vi "NXT Camera Test8.vi"() -> ()   [LabVIEW 2016]
uses:
  <vilib>/NXT/Block Support/NXT_InputPort.ctl
  <vilib>/NXT/Block Support/NXT_OutputPort.ctl
  <vilib>/NXT/Dual Mode Library/Sensors/EV3_Ultrasonic_CM.vi
  <vilib>/NXT/NXTIO Xnodes/NXTIONodeSubVIs/NXTMoveMotors.vi
  <vilib>/NXT/NXTIO Xnodes/NXTIONodeSubVIs/NXTStopMotors.vi
  <vilib>/NXT/Subs/LVHSConnector.ctl
  <vilib>/NXT/NXTIO Xnodes/AddressXNode/NXTIOAddress.xnode
  <vilib>/NXT/NXTIO Xnodes/NXTIOXNode/NXTIO.xnode
  <vilib>/NXT/LegoClasses/BrickReference/BrickReference.lvclass
panel:
  out "Power":bool
  out "X Upper Left":u8
  out "X Lower Right":u8
  out "Y Lower Right":u8
  out "Y Upper Left":u8
  out "Count":u8
  out "Color":u8
  in  "Cluster":T1 {"Tracking Mode" items=["Disable Tracking", "Get First Object", "Get n th Object", "Enable Tracking", "Sort Objects  by size", "Sort Objects  by Colors", "Illumination on ", "Illumination Off", "Write Colormap", "Read Colormap", "Line tracking mode", "Object Tracking mode"]}
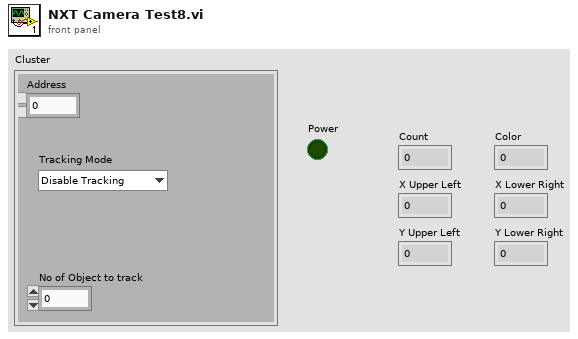
[diagram p1: front panel]
types:
  T1 = cluster{"Address":dbl, "No of Object to track":dbl, "Tracking Mode":u8}
  T2 = cluster{"Tracking Mode":u8, "Object Number to Track":u8, "Address":u8}
  T3 = typedef "NXT_InputPort.ctl" = u32
  T4 = typedef "LVHSConnector.ctl" = refnum<class "BrickReference.lvclass">
  T5 = typedef "NXT_OutputPort.ctl" = u8
  T6 = cluster{"Total Tracked Objects":u8, "Color":u8, "X Upper Left":u8, "Y Upper Left":u8, "X Lower Right":u8, "Y Lower Right":u8, "Status (boolean)":bool}
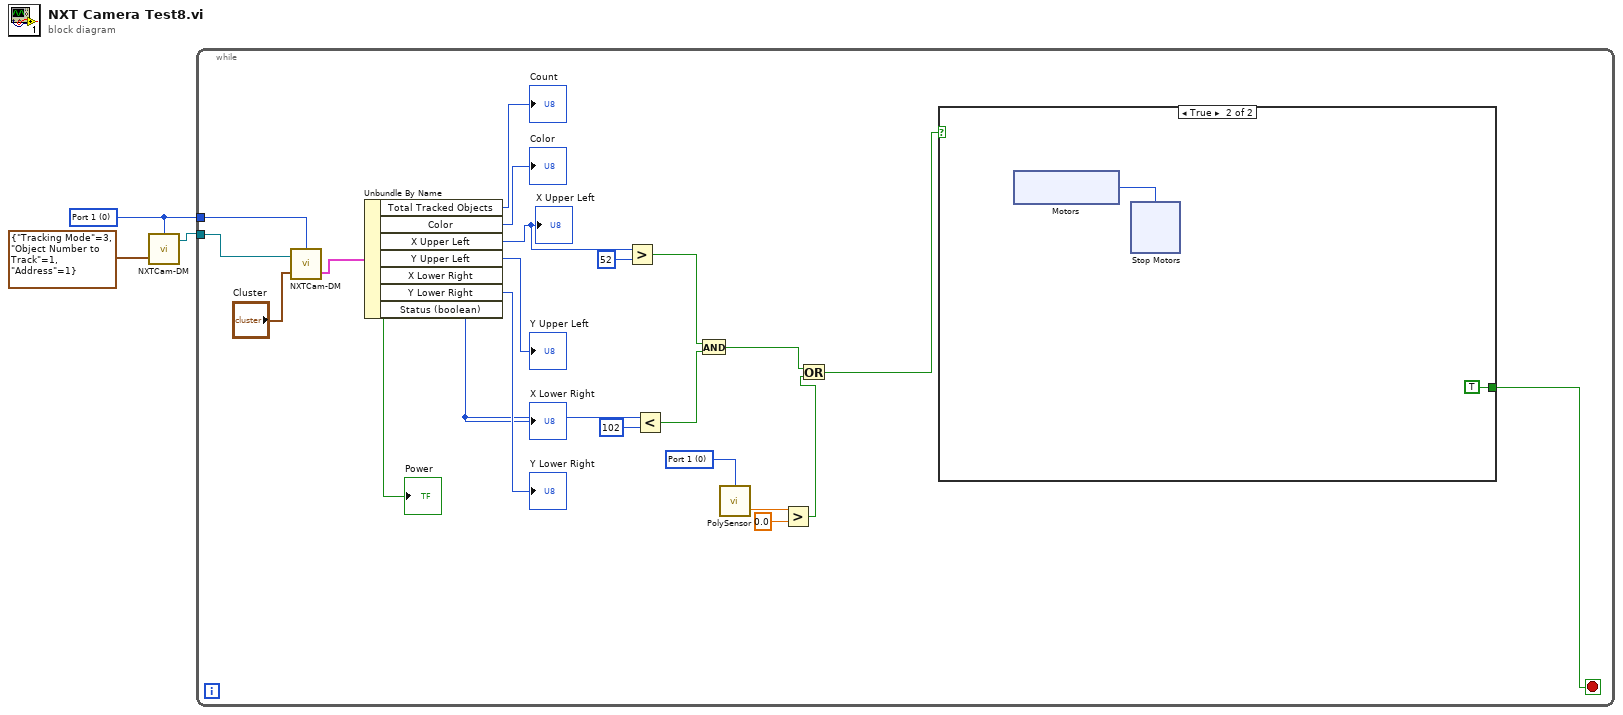
[diagram p0: block diagram]
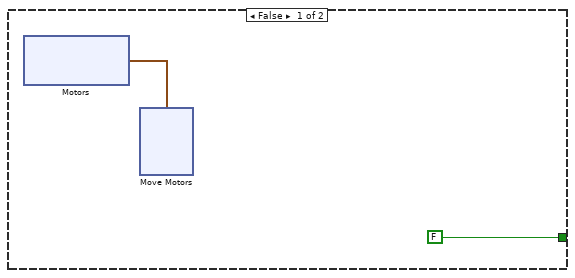
[diagram p2: hidden frame]
diagram:
  w1 = T3 0 items=["Port 1", "Port 2", "Port 3", "Port 4"] ("Input Port")
  n1 = call "NXTCam-DM.vi"("Input of NXTCam"=T2 {"Tracking Mode"=3, "Object Number to Track"=1, "Address"=1}, "Input Port"=w1) -> ("NXT dup"=w3:T4)  [unwired: 1 in, 1 out]
  n2 = while {
    tunnel: w1 -> [w23]
    tunnel: w3 -> [w22]
    stop <- w4 stop-if-true
    w5 = T3 0 items=["Port 1", "Port 2", "Port 3", "Port 4"] ("Port (Port 1)")
    n3 = call "NXTCam-DM.vi"("Input of NXTCam"="Cluster", "NXT"=w22, "Input Port"=w23) -> ("Output of NXTCam"=w18:T6)  [unwired: 1 out]
    n4 = Unbundle By Name(w18) -> ("Total Tracked Objects"=→"Count":u8, "Color"=→"Color":u8, "X Upper Left"=w16:u8, "Y Upper Left"=→"Y Upper Left":u8, "X Lower Right"=w14:u8, "Y Lower Right"=→"Y Lower Right":u8, "Status (boolean)"=→"Power":bool)
    "X Upper Left" <- w16
    "X Lower Right" <- w14
    n5 = Greater?(x=w16, y=u8 52) -> (0:w12:bool)
    n6 = Less?(x=w14, y=u8 102) -> (x < y?=w11:bool)
    n7 = And(x=w12, y=w11) -> (x .and. y?=w8:bool)
    n8 = call-poly <vilib>:"PolySensor.vi"("Port (Port 1)"=w5) -> ("Centimeters"=w10:sgl)  [unwired: 2 in, 1 out]
    n9 = Greater?(x=w10, y=sgl 0.0) -> (0:w7:bool)
    n10 = Or(x=w8, y=w7) -> (x .or. y?=w6:bool)
    n11 = case shown="True" w6 {
      tunnel: [FALSE TRUE] -> w4
      frame False {
        n12 = xnode "Motors"() -> ("Motor"=w27:cluster{"Port":T5, "Port":T5})
        n13 = xnode "Move Motors"("Motors"=w27) -> ()  [unwired: 3 in, 1 out]
      }
      frame True {
        n14 = xnode "Motors"() -> ("Motor"=w38:T5)
        n15 = xnode "Stop Motors"("Motors"=w38) -> ()  [unwired: 1 in, 1 out]
      }
    }
  }
